vi "Lock Controls.vi"(8 "error in (no error)":errorcluster, 10 "Lock Controls?":bool, 11 "MSOX6004 in":refnum<class "MSOX6004.lvclass">) -> (0 "error out":errorcluster, 3 "MSOX6004 out":refnum<class "MSOX6004.lvclass">)   [LabVIEW 2018, in "MSOX6004.lvlib" / "MSOX6004.lvclass"]
doc: "This override method is used to lock/unlock user access to the oscilloscope front panel controls."
uses:
  MSOX6004.lvclass
  MSOX6004.lvclass/MSOX6004.ctl
  <instrlib>/Keysight InfiniiVision/Keysight InfiniiVision.lvlib
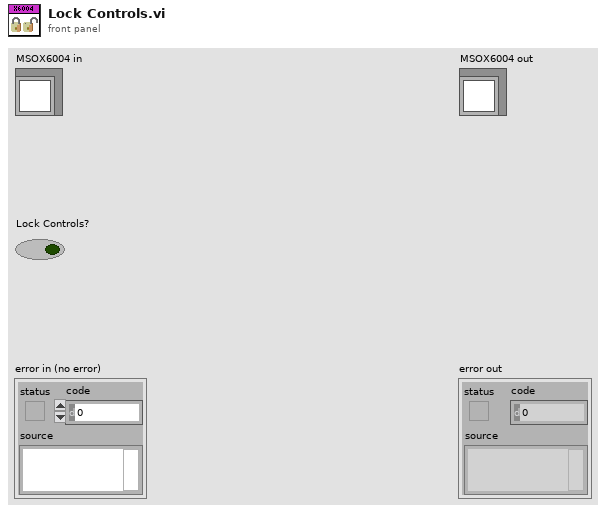
[diagram p1: front panel]
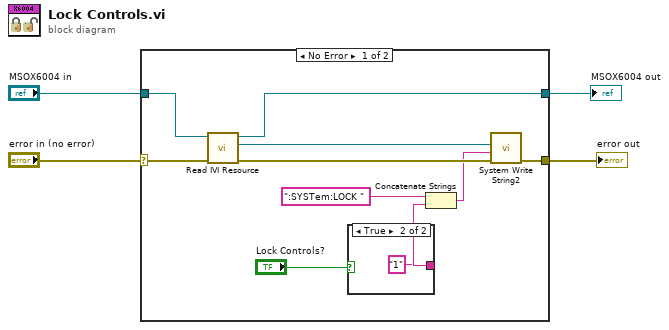
[diagram p0: block diagram]
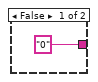
[diagram p2: hidden frame]
diagram:
  n1 = case shown="No Error" "error in (no error)" {
    selector: "error in (no error)" -> [w14 w18]
    tunnel: [w7 w18] -> w3
    tunnel: [w12 w17] -> w2
    tunnel: "MSOX6004 in" -> [w13 w17]
    frame No Error {
      n2 = call "Read IVI Resource.vi"("error in (no error)"=w14, "MSOX6004 in"=w13) -> ("error out"=w8:errorcluster, "IVI Resource"=w6:refnum<k15>, "MSOX6004 out"=w12:refnum<class "MSOX6004.lvclass">)  [unwired: 7 in]
      n3 = case shown="True" "Lock Controls?" {
        tunnel: ["0" "1"] -> w9
        frame False {
        }
        frame True {
        }
      }
      n4 = Concatenate Strings(":SYSTem:LOCK ", w9) -> (w5:string)
      n5 = call <instrlib>:"System Write String2.vi"("error in (no error)"=w8, "Data"=w5, "instrument handle"=w6) -> ("error out"=w7:errorcluster)  [unwired: 7 in, 1 out]
    }
    frame Error {
    }
  }
  "error out" <- w3
  "MSOX6004 out" <- w2
